vi "_INIT_COS_LUT_2048.vi"() -> (0 "Init Data Out":u16[](array[numeric]))   [LabVIEW 2018]
panel:
  # "For Initialization VI requirements and help, please read directions located on Block Diagram."
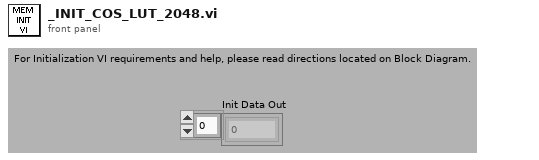
[diagram p1: front panel]
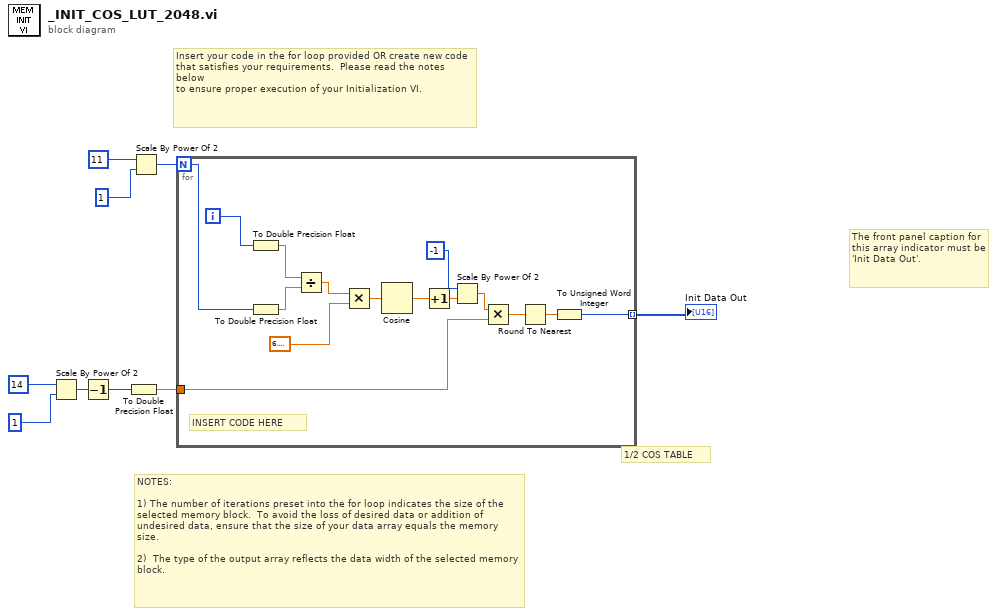
[diagram p0: block diagram]
diagram:
  # "1/2 COS TABLE"
  # "The front panel caption for this array indicator must be 'Init Data Out'."
  # "NOTES:\n\n1) The number of iterations preset into the for loop indicates the size of the selected memory block.  To avoid the loss of desired data or addition of undesired data, ensure that the size of your data array equals the memory size.\n\n2)  The type of the output array reflects the data width of the selected memory block."
  # "Insert your code in the for loop provided OR create new code\nthat satisfies your requirements.  Please read the notes below\nto ensure proper execution of your Initialization VI."
  n1 = Scale By Power Of 2(n=i16 14, x=1) -> (x*2^n=w2:i32)
  n2 = Decrement(x=w2) -> (x-1=w1:i32)
  n3 = To Double Precision Float(number=w1) -> (double precision float=w3:dbl)
  n4 = Scale By Power Of 2(n=i16 11, x=1) -> (x*2^n=w6:i32)
  n5 = for {
    N: w6 -> [w23]
    tunnel: [w12] -> w9 mode=indexing
    tunnel: w3 -> [w16]
    i -> [w24]
    # "INSERT CODE HERE"
    n6 = To Double Precision Float(number=w24) -> (double precision float=w22:dbl)
    n7 = To Double Precision Float(number=w23) -> (double precision float=w21:dbl)
    n8 = Divide(x=w22, y=w21) -> (x/y=w20:dbl)
    n9 = Multiply(x=w20, y=6.283185307179586) -> (x*y=w19:dbl)
    n10 = Cosine(x=w19) -> (cos(x)=w17:dbl)
    n11 = Increment(x=w17) -> (x+1=w15:dbl)
    n12 = Scale By Power Of 2(n=i16 -1, x=w15) -> (x*2^n=w11:dbl)
    n13 = Multiply(x=w11, y=w16) -> (x*y=w14:dbl)
    n14 = Round To Nearest(number=w14) -> (nearest integer value=w13:dbl)
    n15 = To Unsigned Word Integer(number=w13) -> (unsigned 16bit integer=w12:u16)
  }
  "Init Data Out" <- w9
